vi "Page_Source_Send_To_MainDest_OnAdd.vi"(8 "error in (no error)":errorcluster, 11 "AB_Build in":refnum<class "AB_Build.lvclass">) -> (0 "error out":errorcluster, 2 "send to main dest":bool, 3 "AB_Build out":refnum<class "AB_Build.lvclass">)   [LabVIEW 2020, in "AB_Build.lvclass"]
uses:
  <vilib>/AppBuilder/AB_Classes/Build/AB_Build.lvclass
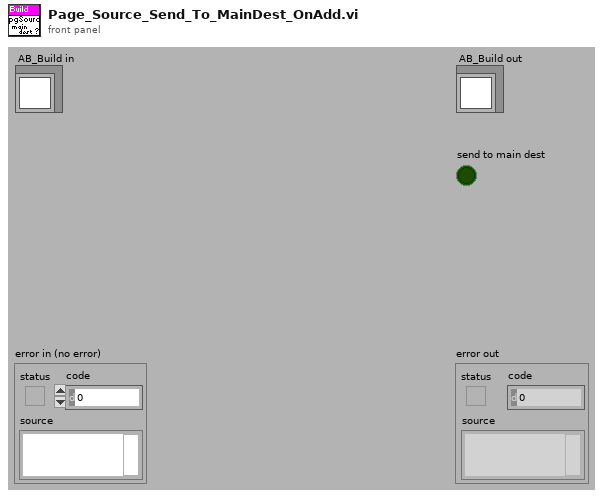
[diagram p1: front panel]
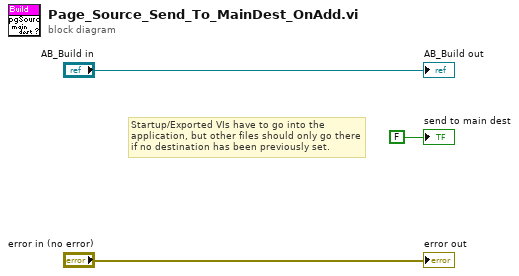
[diagram p0: block diagram]
diagram:
  # "Startup/Exported VIs have to go into the application, but other files should only go there if no destination has been previously set."
  "error out" <- "error in (no error)"
  "AB_Build out" <- "AB_Build in"
  "send to main dest" <- FALSE ("canAddToTop")
